vi "To String.vi"(8 "error in (no error)":errorcluster, 11 "Generic Data in":refnum<class "Generic Data.lvclass">) -> (0 "error out":errorcluster, 2 "String":string)   [LabVIEW 2020, in "Data.lvlib" / "Generic Data.lvclass"]
doc: "Convert 'Generic Data in' to a string.\nThe default implementation convert the data to an XML string."
uses:
  Generic Data.lvclass
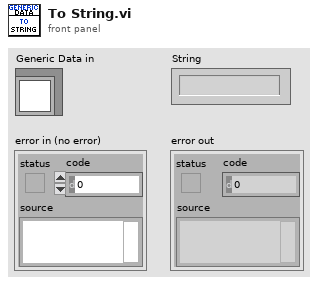
[diagram p1: front panel]
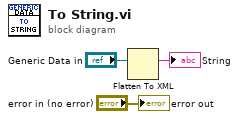
[diagram p0: block diagram]
diagram:
  n1 = Flatten To XML(6:"Generic Data in") -> (2:→"String":string)
  "error out" <- "error in (no error)"
